vi "Main ACQ module2.vi"(8 "Update timer[ms]":u32=100, 9 "Master mailbox":T6, 11 "Module mailbox":T6) -> ()   [LabVIEW 2024, in "Lock-in module.lvlib"]
uses:
  Lock-in module.lvlib
  Messenger service/Data types/Mailbox address.ctl
  ctl/ACQ status.ctl
  <instrlib>/Zurich Instruments LabOne/Public/ziTypeHandle.ctl
  <instrlib>/Zurich Instruments LabOne/Public/Modules/ziTypeModHandle.ctl
  ctl/ACQ info.ctl
  ctl/Mode.ctl
  Messenger service/Data types/Module name.ctl
  ctl/MFLI_message for module.ctl
  ctl/MFLI_command enum.ctl
  ctl/MFLI parameters.ctl
  <instrlib>/Zurich Instruments LabOne/Public/Modules/ziTypeModEnum.ctl
  ctl/MFLI_parameter and value.ctl
  ctl/MFLI_node.ctl
  <instrlib>/Zurich Instruments LabOne/Public/Configure/ziSetValueDouble.vi
  <instrlib>/Zurich Instruments LabOne/Zurich Instruments LabOne.lvlib
  Messenger service/MessengerLib.lvlib
panel:
  out "time":u32
  out "Modulation amplitude [A]":dbl
  out "Multimeter name":string
  out "Multimeter port":refnum<visa-resource-name>
  out "Mode":T1=enum."Point"
  out "ACQ  status":T2={"Lock-in Handle"={"handleValid"=FALSE, "Conn"=0, "Path Prefix"="", "Handle"=0, "Connected"=FALSE, "Clockbase(s)"=0.0}, "Address"="DEV", "ModuleHandles"=[], "Lock-in info"={"In50"=FALSE, "InAC"=FALSE, "InDiff"=FALSE, "Out50"=FALSE, "OutEN"=FALSE, "OutF[Hz]"=0.0, "OutA[V]"=0.0, "DemEN"=FALSE, "Const[ms]"=0.0, "Order[-]"=0, "Phase [°]"=0.0}} {"ModuleHandles"."ModHandle" format="0x%08x"; "ModuleHandles"."Conn" format="0x%08x"; "Lock-in Handle"."Handle" format="0x%08x"; "Lock-in Handle"."Conn" format="0x%08x"}
  out "Selected Device":string
  out "Ended":bool
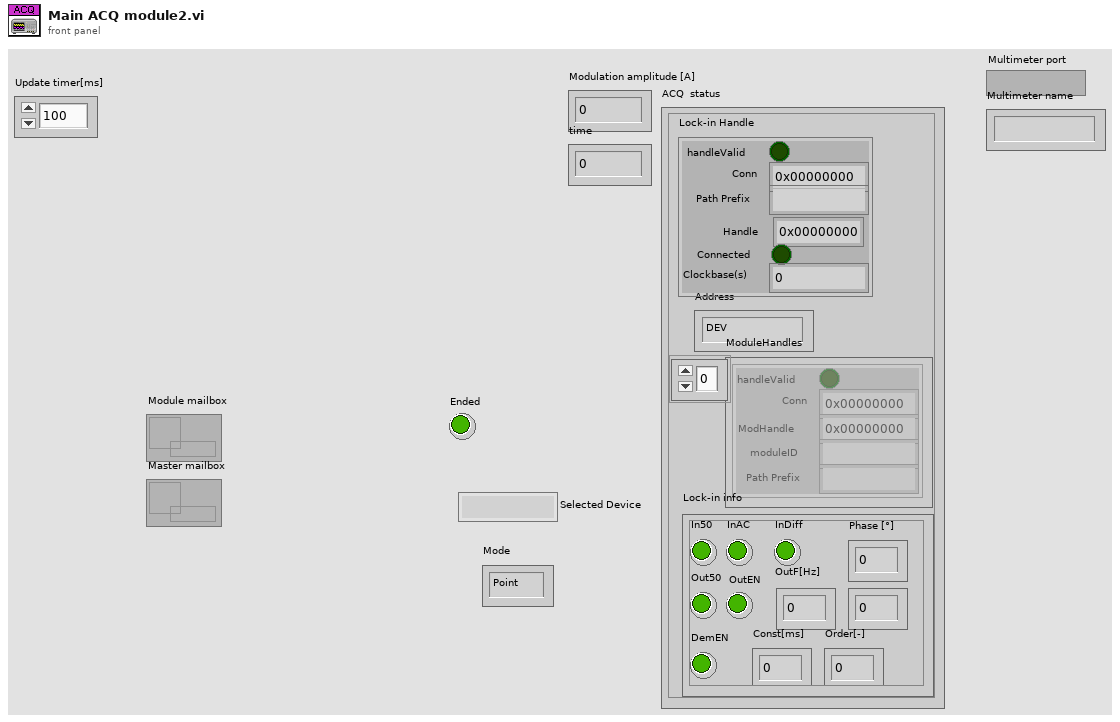
[diagram p1: front panel]
types:
  T1 = typedef "Lock-in module.lvlib/Mode.ctl" = enum16{"None", "Point", "Scope", "Both", "DAQ"}
  T2 = typedef "Lock-in module.lvlib/ACQ status.ctl" = cluster{"Lock-in Handle":T3, "Address":string, "ModuleHandles":T4[], "Lock-in info":T5}
  T3 = typedef "Zurich Instruments LabOne.lvlib/ziTypeHandle.ctl" = cluster{"handleValid":bool, "Conn":u64, "Path Prefix":string, "Handle":u64, "Connected":bool, "Clockbase(s)":dbl}
  T4 = typedef "Zurich Instruments LabOne.lvlib/ziTypeModHandle.ctl" = cluster{"handleValid":bool, "Conn":u64, "ModHandle":u64, "moduleID":string, "Path Prefix":string}
  T5 = typedef "Lock-in module.lvlib/ACQ info.ctl" = cluster{"In50":bool, "InAC":bool, "InDiff":bool, "Out50":bool, "OutEN":bool, "OutF[Hz]":dbl, "OutA[V]":dbl, "DemEN":bool, "Const[ms]":dbl, "Order[-]":i32, "Phase [°]":dbl}
  T6 = typedef "MessengerLib.lvlib/Mailbox address.ctl" = refnum<queue>
  T7 = typedef "Module name.ctl" = enum16{"Emty", "Magnet", "VTI", "Excitation", "Servo", "Acquisition", "Rotator", "Digitizer", "SMU2450", "Carousel", "Multimeter", "Tmp monitor", "Power monitor"}
  T8 = typedef "Lock-in module.lvlib/MFLI parameters.ctl" = cluster{"Filter order":dbl, "Time constant [ms]":dbl, "F_Mod [kHz]":dbl, "Amp_Mod [mV]":dbl, "Enable output":u16, "Phase [°]":dbl}
  T9 = typedef "Lock-in module.lvlib/MFLI_parameter and value.ctl" = cluster{"parameter":T10, "value":dbl}
  T10 = typedef "Lock-in module.lvlib/MFLI_node.ctl" = enum16{"None", "filter_order [-]", "filter_constant [ms]", "in_diff", "in_autorange", "in_imp50", "in_AC", "osc_freq [kHz]", "out_ampl [V]", "out_autorange", "out_imp50", "enable output", "enamble ampl", "scope_enable", "scope_rate", "scope_len", "scope_trigEn", "AuxOut_amplify", "Phase_deg", "AuxOut_select"}
  T11 = typedef "Lock-in module.lvlib/MFLI_command enum.ctl" = enum16{"Initialize", "Update", "Set parameters", "Set module", "Set individual parameters", "Get point", "Get array", "Disconnect", "End", "Ignore"}
  T12 = typedef "Zurich Instruments LabOne.lvlib/ziTypeModEnum.ctl" = u16
  T13 = typedef "Lock-in module.lvlib/MFLI_message for module.ctl" = cluster{"Command":T11, "Data":variant}
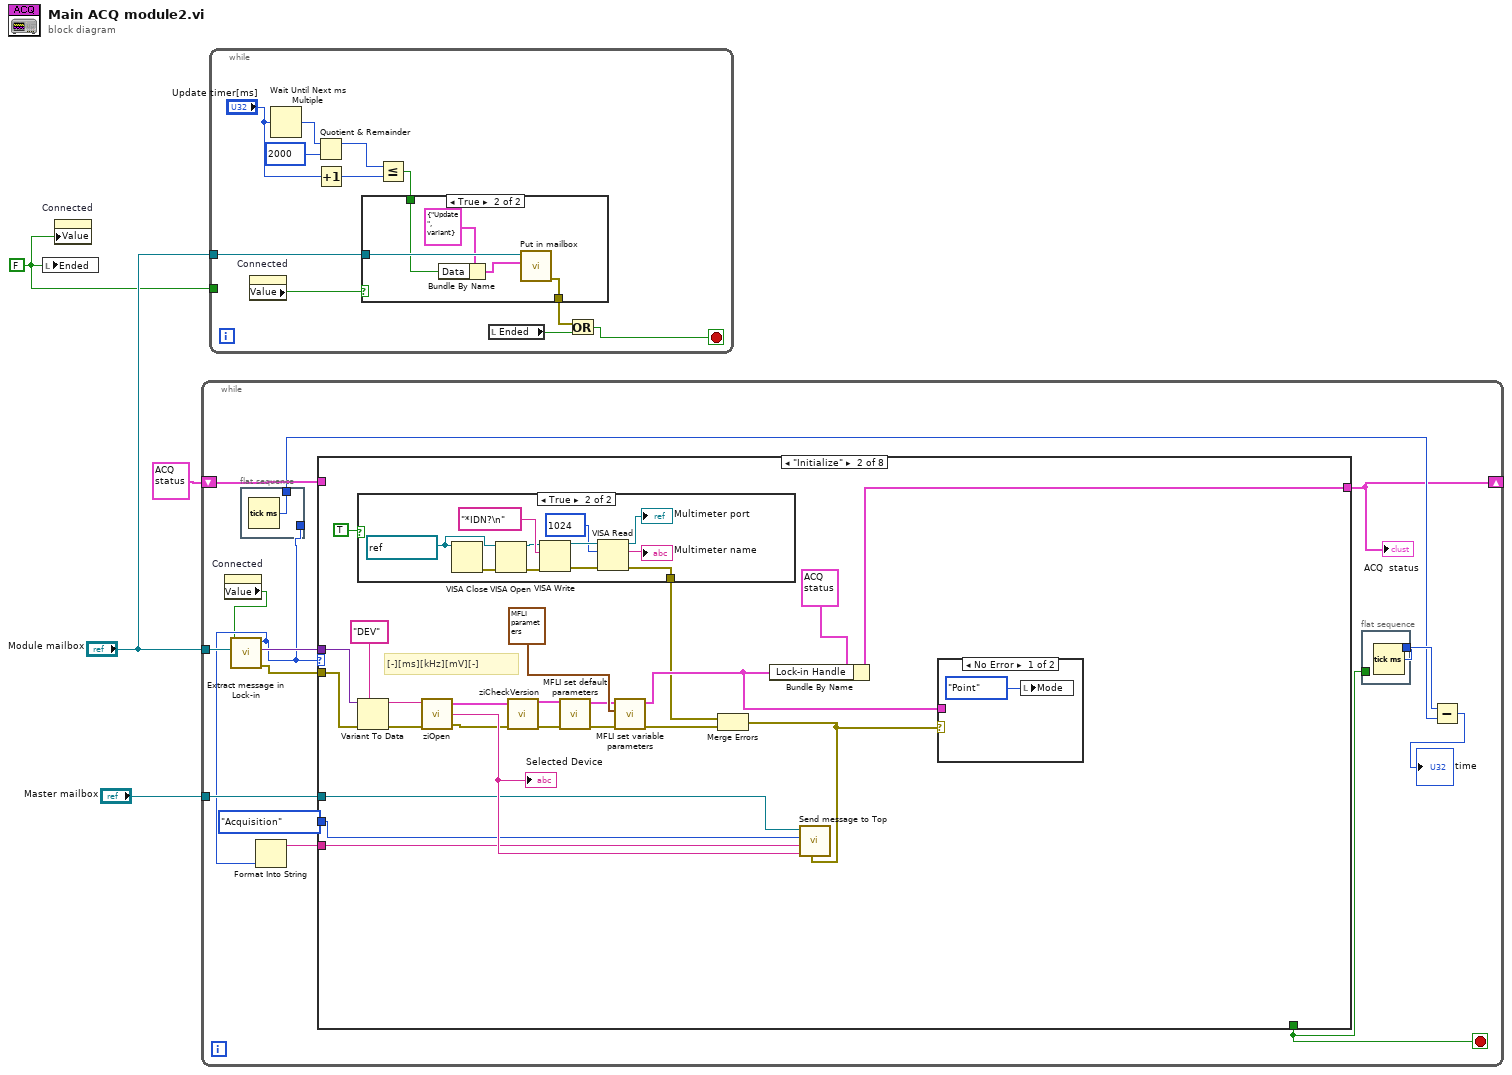
[diagram p0: block diagram]
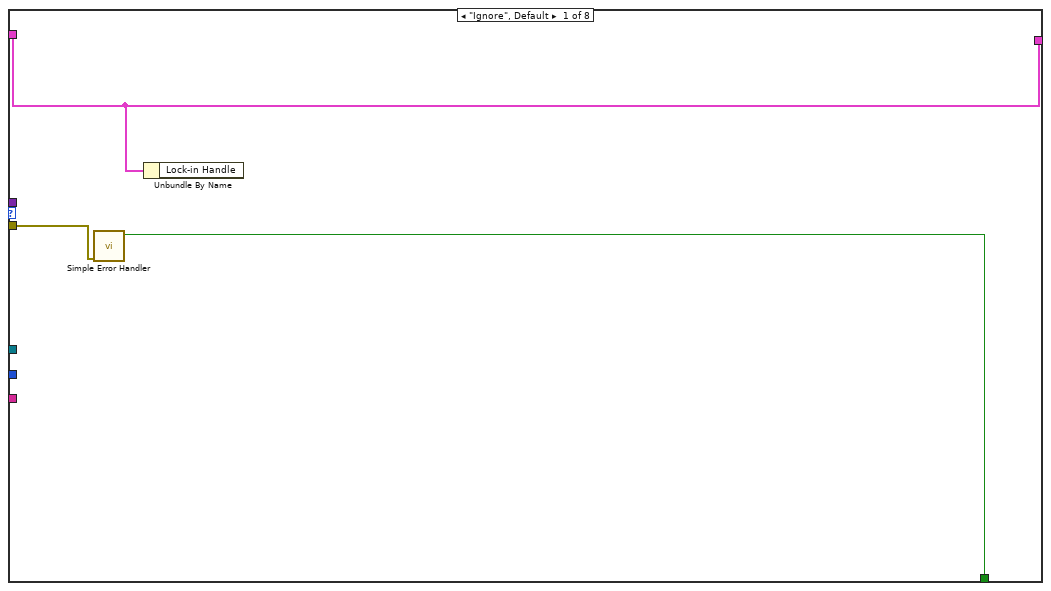
[diagram p2: hidden frame]
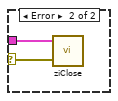
[diagram p4: hidden frame]
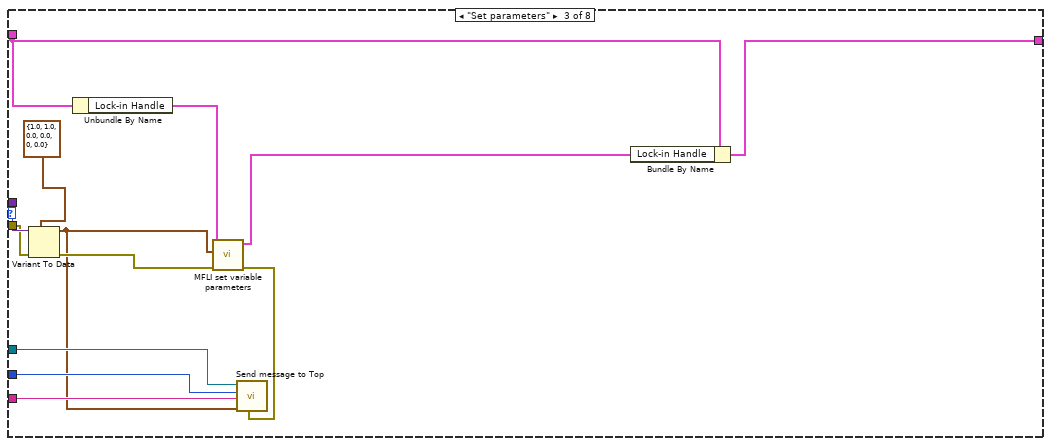
[diagram p5: hidden frame]
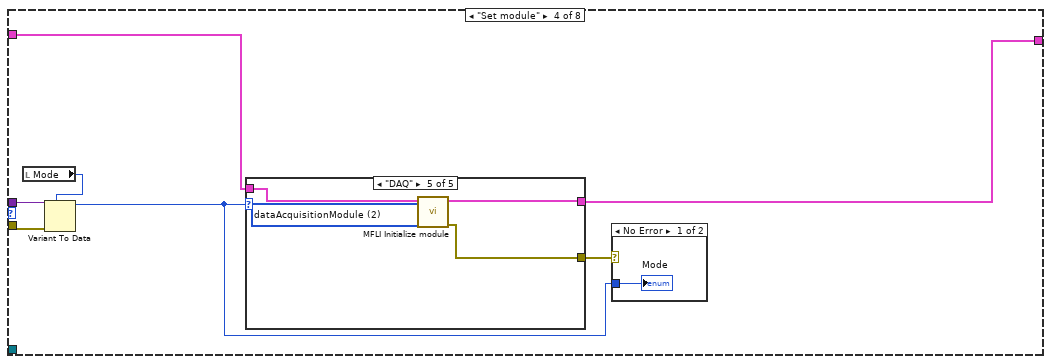
[diagram p6: hidden frame]
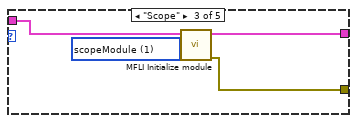
[diagram p10: hidden frame]
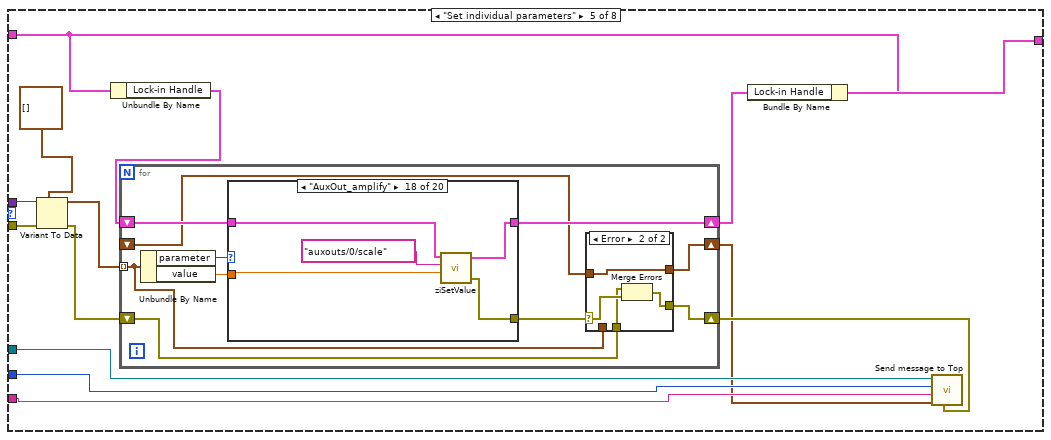
[diagram p12: hidden frame]
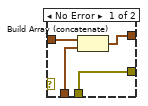
[diagram p13: hidden frame]
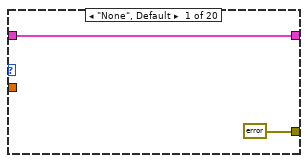
[diagram p14: hidden frame]
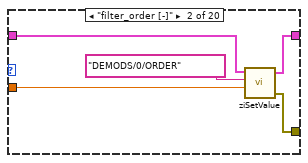
[diagram p15: hidden frame]
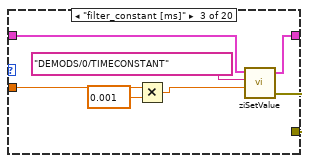
[diagram p16: hidden frame]
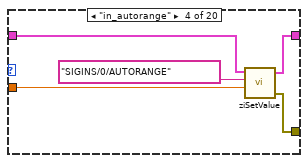
[diagram p17: hidden frame]
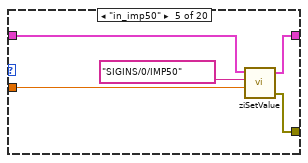
[diagram p18: hidden frame]
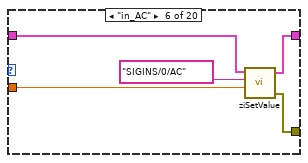
[diagram p19: hidden frame]
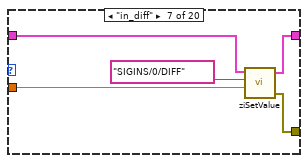
[diagram p20: hidden frame]
diagram:
  w1 = FALSE ("Initialized")
  n1 = local write "Ended"(w1) -> ()
  n2 = property on="Connected" class="Bool (strict)"("Value"=w1) -> ()  [unwired: 2 in, 2 out]
  n3 = while {
    tunnel: "Module mailbox" -> [w18]
    tunnel: "Master mailbox" -> [w17]
    shift-right: [w7] -> _
    shift-left: T2 {"Lock-in Handle"={"handleValid"=FALSE, "Conn"=0, "Path Prefix"="", "Handle"=0, "Connected"=FALSE, "Clockbase(s)"=0.0}, "Address"="DEV", "ModuleHandles"=[], "Lock-in info"={"In50"=FALSE, "InAC"=FALSE, "InDiff"=FALSE, "Out50"=FALSE, "OutEN"=FALSE, "OutF[Hz]"=0.0, "OutA[V]"=0.0, "DemEN"=FALSE, "Const[ms]"=0.0, "Order[-]"=0, "Phase [°]"=0.0}} -> [w14]
    stop <- w6 stop-if-true
    n4 = property on="Connected" class="Bool (strict)"() -> ("Value"=w5:bool)  [unwired: 2 in, 2 out]
    n5 = call "Extract message in Lock-in.vi"("Module mailbox"=w18, "Initialized?"=w5) -> ("error out"=w15:errorcluster, "Data"=w16:variant, "Command out"=w11:T11)  [unwired: 7 in]
    n6 = flat-sequence {
      tunnel: w11 -> [_]
      tunnel: [w20] -> w9
      frame #0 {
        n7 = Tick Count (ms)() -> (millisecond timer value=w20:u32)
      }
    }
    n8 = Format Into String(w11) -> (resulting string=w13:string)  [unwired: 3 in, 1 out]
    n9 = case shown="\"Initialize\"" w11 {
      tunnel: w17 -> [_ w39 w68 _ w96 w239 w283 w300]
      tunnel: w16 -> [_ w46 w73 w80 w106 w231 _ _]
      tunnel: w15 -> [w23 w44 w69 w79 w104 w243 w284 w301]
      tunnel: [w22 _ _ _ _ _ w274 FALSE] -> w6
      tunnel: [w21 w38 w70 w76 w103 w245 w276 w292] -> w7
      tunnel: w14 -> [w21 _ w71 w77 w101 w237 w285 w302]
      tunnel: w13 -> [_ w35 w67 _ w98 w234 w281 w297]
      tunnel: Module_name."Acquisition" ("Module") -> [_ w34 w66 _ w97 w236 w282 w298]
      frame "Ignore", Default {
        n10 = call <vilib>:"Simple Error Handler.vi"("error in (no error)"=w23) -> ("error?"=w22:bool)  [unwired: 4 in, 4 out]
        n11 = Unbundle By Name(w21) -> ()  [unwired: 1 out]
      }
      frame "Initialize" {
        # "[-][ms][kHz][mV][-]"
        n12 = case shown="True" TRUE {
          tunnel: [_ w49] -> w25
          frame False {
          }
          frame True {
            w56 = refnum<visa-resource-name> "COM6" ("VISA resource name")
            n13 = VISA Close(VISA resource name=w56) -> (error out=w57:errorcluster)  [unwired: 1 in]
            n14 = VISA Open(error in (no error)=w57, VISA resource name=w56) -> (VISA resource name=w51:refnum<visa-resource-name>, error out=w50:errorcluster)  [unwired: 3 in]
            n15 = VISA Write(VISA resource name=w51, write buffer="*IDN?\n", error in (no error)=w50) -> (VISA resource name out=w55:refnum<visa-resource-name>, error out=w54:errorcluster)  [unwired: 1 out]
            n16 = VISA Read(VISA resource name=w55, byte count=u32 1024, error in (no error)=w54) -> (VISA resource name out=→"Multimeter port":refnum<visa-resource-name>, read buffer=→"Multimeter name":string, error out=w49:errorcluster)  [unwired: 1 out]
          }
        }
        n17 = Variant To Data(error in=w44, type="DEV" ("Address"), Variant=w46) -> (data=w43:string, error out=w42:errorcluster)
        n18 = call <instrlib>:"ziOpen.vi"("Error In"=w42, "Address"=w43) -> ("Error Out"=w36:errorcluster, "Selected Device"=w40:string, "HandleOut"=w37:T3)  [unwired: 2 in]
        "Selected Device" <- w40
        n19 = call <instrlib>:"ziCheckVersion.vi"("Handle In"=w37, "Error In"=w36) -> ("Handle Out"=w32:T3, "Error Out"=w33:errorcluster)  [unwired: 11 in, 1 out]
        n20 = call "MFLI set default parameters.vi"("error in (no error)"=w33, "Lock-in Handle"=w32) -> ("Error Out"=w29:errorcluster, "Handle Out"=w30:T3)  [unwired: 8 in]
        n21 = call "MFLI set variable parameters.vi"("error in"=w29, "ACQ parameters"=T8 {"Filter order"=5.0, "Time constant [ms]"=50.0, "F_Mod [kHz]"=10.0, "Amp_Mod [mV]"=100.0, "Enable output"=0, "Phase [°]"=0.0}, "handle in"=w30) -> ("Error Out"=w28:errorcluster, "Handle Out"=w26:T3)  [unwired: 7 in]
        n22 = Merge Errors(w25, w28) -> (w27:errorcluster)
        n23 = Bundle By Name(cluster=T2 {"Lock-in Handle"={"handleValid"=FALSE, "Conn"=0, "Path Prefix"="", "Handle"=0, "Connected"=FALSE, "Clockbase(s)"=0.0}, "Address"="DEV", "ModuleHandles"=[], "Lock-in info"={"In50"=FALSE, "InAC"=FALSE, "InDiff"=FALSE, "Out50"=FALSE, "OutEN"=FALSE, "OutF[Hz]"=0.0, "OutA[V]"=0.0, "DemEN"=FALSE, "Const[ms]"=0.0, "Order[-]"=0, "Phase [°]"=0.0}}, "Lock-in Handle"=w26) -> (w38:T2)
        n24 = call "Send message to Top.vi"("Error in (no error)"=w27, "Data"=w40, "Response"=w35, "Module"=w34, "Mailbox address in"=w39) -> ()  [unwired: 5 in, 2 out]
        n25 = case shown="No Error" w27 {
          selector: w27 -> [_ w60]
          tunnel: w26 -> [_ w59]
          frame No Error {
            n26 = local write "Mode"(Mode."Point" ("Mode")) -> ()
          }
          frame Error {
            n27 = call <instrlib>:"ziClose.vi"("Error In"=w60, "Handle In"=w59) -> ()  [unwired: 2 in, 2 out]
          }
        }
      }
      frame "Set parameters" {
        n28 = Variant To Data(error in=w69, type=T8 {"Filter order"=1.0, "Time constant [ms]"=1.0, "F_Mod [kHz]"=0.0, "Amp_Mod [mV]"=0.0, "Enable output"=0, "Phase [°]"=0.0} ("ACQ parameters"), Variant=w73) -> (data=w61:T8, error out=w63:errorcluster)
        n29 = Unbundle By Name(w71) -> ("Lock-in Handle"=w64:T3)
        n30 = call "MFLI set variable parameters.vi"("error in"=w63, "ACQ parameters"=w61, "handle in"=w64) -> ("Error Out"=w65:errorcluster, "Handle Out"=w62:T3)  [unwired: 7 in]
        n31 = call "Send message to Top.vi"("Error in (no error)"=w65, "Data"=w61, "Response"=w67, "Module"=w66, "Mailbox address in"=w68) -> ()  [unwired: 5 in, 2 out]
        n32 = Bundle By Name(cluster=w71, "Lock-in Handle"=w62) -> (w70:T2)
      }
      frame "Set module" {
        n33 = local read "Mode"() -> (w78:T1)
        n34 = Variant To Data(error in=w79, type=w78, Variant=w80) -> (data=w74:T1)  [unwired: 1 out]
        n35 = case shown="\"DAQ\"" w74 {
          tunnel: w77 -> [w82 w83 w86 w88 w92]
          tunnel: [w82 w83 w85 w88 w90] -> w76
          tunnel: [_ _ w84 _ w89] -> w75
          frame "None", Default {
          }
          frame "Point" {
          }
          frame "Scope" {
            w87 = T12 1 items=["sweep", "scopeModule", "dataAcquisitionModule", "pidAdvisor", "awgModule", "impedanceModule", "multiDeviceSyncModule", "zoomFFT", "trigger", "deviceSettings", "record"] ("module Id")
            n36 = call "MFLI Initialize module.vi"("module Id"=w87, "ACQ  status in"=w86) -> ("Error Out"=w84:errorcluster, "ACQ  status out"=w85:T2)  [unwired: 8 in]
          }
          frame "Both" {
          }
          frame "DAQ" {
            w91 = T12 2 items=["sweep", "scopeModule", "dataAcquisitionModule", "pidAdvisor", "awgModule", "impedanceModule", "multiDeviceSyncModule", "zoomFFT", "trigger", "deviceSettings", "record"] ("module Id")
            n37 = call "MFLI Initialize module.vi"("module Id"=w91, "ACQ  status in"=w92) -> ("Error Out"=w89:errorcluster, "ACQ  status out"=w90:T2)  [unwired: 8 in]
          }
        }
        n38 = case shown="No Error" w75 {
          tunnel: w74 -> [w81 _]
          frame No Error {
            "Mode" <- w81
          }
          frame Error {
          }
        }
      }
      frame "Set individual parameters" {
        n39 = Variant To Data(error in=w104, type=T9[] [] ("Array"), Variant=w106) -> (data=w99:T9[], error out=w94:errorcluster)
        n40 = Unbundle By Name(w101) -> ("Lock-in Handle"=w102:T3)
        n41 = for {
          tunnel: w99 -> [w109] mode=indexing
          shift-right: [w115] -> w100
          shift-left: w102 -> [w116]
          shift-right: [w111] -> w95
          shift-left: w94 -> [w110]
          shift-right: [w108] -> w93
          shift-left: _ -> [w107]
          n42 = Unbundle By Name(w109) -> ("parameter"=w113:T10, "value"=w114:dbl)
          n43 = case shown="\"AuxOut_amplify\"" w113 {
            tunnel: w116 -> [w126 w131 w138 w143 w148 w153 w158 w165 w170 w175 w180 w185 w190 w195 w198 w205 w208 w213 w218 w223]
            tunnel: [w126 w130 w137 w142 w147 w152 w157 w164 w169 w174 w179 w184 w189 w194 w199 w204 w209 w214 w219 w224] -> w115
            tunnel: w114 -> [_ w129 w136 w141 w146 w151 w156 w161 w168 w173 w178 w183 w188 w192 w197 w203 w207 w212 w217 w222]
            tunnel: [errorcluster {"status"=FALSE, "code"=0, "source"=""} ("Error Out") w127 w134 w139 w144 w149 w154 w163 w166 w171 w176 w181 w186 w193 w200 w201 w210 w215 w220 w225] -> w112
            frame "None", Default {
            }
            frame "filter_order [-]" {
              n44 = call-poly <instrlib>:"ziSetValue.vi"("Value"=w129, "Path"="DEMODS/0/ORDER", "Handle In"=w131) -> ("Error Out"=w127:errorcluster, "Handle Out"=w130:T3)  [unwired: 2 in]
            }
            frame "filter_constant [ms]" {
              n45 = Multiply(x=w136, y=0.001) -> (x*y=w133:dbl)
              n46 = call-poly <instrlib>:"ziSetValue.vi"("Value"=w133, "Path"="DEMODS/0/TIMECONSTANT", "Handle In"=w138) -> ("Error Out"=w134:errorcluster, "Handle Out"=w137:T3)  [unwired: 2 in]
            }
            frame "in_autorange" {
              n47 = call-poly <instrlib>:"ziSetValue.vi"("Value"=w141, "Path"="SIGINS/0/AUTORANGE", "Handle In"=w143) -> ("Error Out"=w139:errorcluster, "Handle Out"=w142:T3)  [unwired: 2 in]
            }
            frame "in_imp50" {
              n48 = call-poly <instrlib>:"ziSetValue.vi"("Value"=w146, "Path"="SIGINS/0/IMP50", "Handle In"=w148) -> ("Error Out"=w144:errorcluster, "Handle Out"=w147:T3)  [unwired: 2 in]
            }
            frame "in_AC" {
              n49 = call-poly <instrlib>:"ziSetValue.vi"("Value"=w151, "Path"="SIGINS/0/AC", "Handle In"=w153) -> ("Error Out"=w149:errorcluster, "Handle Out"=w152:T3)  [unwired: 2 in]
            }
            frame "in_diff" {
              n50 = call-poly <instrlib>:"ziSetValue.vi"("Value"=w156, "Path"="SIGINS/0/DIFF", "Handle In"=w158) -> ("Error Out"=w154:errorcluster, "Handle Out"=w157:T3)  [unwired: 2 in]
            }
            frame "osc_freq [kHz]" {
              n51 = Multiply(x=w161, y=1000.0) -> (x*y=w160:dbl)
              n52 = call-poly <instrlib>:"ziSetValue.vi"("Value"=w160, "Path"="OSCS/0/FREQ", "Handle In"=w165) -> ("Error Out"=w163:errorcluster, "Handle Out"=w164:T3)  [unwired: 2 in]
            }
            frame "out_ampl [V]" {
              n53 = call-poly <instrlib>:"ziSetValue.vi"("Value"=w168, "Path"="SIGOUTS/0/AMPLITUDES/1", "Handle In"=w170) -> ("Error Out"=w166:errorcluster, "Handle Out"=w169:T3)  [unwired: 2 in]
            }
            frame "out_autorange" {
              n54 = call-poly <instrlib>:"ziSetValue.vi"("Value"=w173, "Path"="SIGOUTS/0/AUTORANGE", "Handle In"=w175) -> ("Error Out"=w171:errorcluster, "Handle Out"=w174:T3)  [unwired: 2 in]
            }
            frame "out_imp50" {
              n55 = call-poly <instrlib>:"ziSetValue.vi"("Value"=w178, "Path"="SIGOUTS/0/IMP50", "Handle In"=w180) -> ("Error Out"=w176:errorcluster, "Handle Out"=w179:T3)  [unwired: 2 in]
            }
            frame "enable output" {
              n56 = call-poly <instrlib>:"ziSetValue.vi"("Value"=w183, "Path"="SIGOUTS/0/ON", "Handle In"=w185) -> ("Error Out"=w181:errorcluster, "Handle Out"=w184:T3)  [unwired: 2 in]
            }
            frame "enamble ampl" {
              n57 = call-poly <instrlib>:"ziSetValue.vi"("Value"=w188, "Path"="SIGOUTS/0/ENABLES/1", "Handle In"=w190) -> ("Error Out"=w186:errorcluster, "Handle Out"=w189:T3)  [unwired: 2 in]
            }
            frame "scope_enable" {
              n58 = call-poly <instrlib>:"ziSetValue.vi"("Value"=w192, "Path"="scopes/0/enable", "Handle In"=w195) -> ("Error Out"=w193:errorcluster, "Handle Out"=w194:T3)  [unwired: 2 in]
            }
            frame "scope_rate" {
              n59 = call-poly <instrlib>:"ziSetValue.vi"("Value"=w197, "Path"="scopes/0/time", "Handle In"=w198) -> ("Error Out"=w200:errorcluster, "Handle Out"=w199:T3)  [unwired: 2 in]
            }
            frame "scope_trigEn" {
              n60 = call-poly <instrlib>:"ziSetValue.vi"("Value"=w203, "Path"="SCOPES/0/TRIGENABLE", "Handle In"=w205) -> ("Error Out"=w201:errorcluster, "Handle Out"=w204:T3)  [unwired: 2 in]
            }
            frame "scope_len" {
              n61 = call-poly <instrlib>:"ziSetValue.vi"("Value"=w207, "Path"="scopes/0/length", "Handle In"=w208) -> ("Error Out"=w210:errorcluster, "Handle Out"=w209:T3)  [unwired: 2 in]
            }
            frame "AuxOut_amplify" {
              n62 = call-poly <instrlib>:"ziSetValue.vi"("Value"=w212, "Path"="auxouts/0/scale", "Handle In"=w213) -> ("Error Out"=w215:errorcluster, "Handle Out"=w214:T3)  [unwired: 2 in]
            }
            frame "Phase_deg" {
              n63 = call-poly <instrlib>:"ziSetValue.vi"("Value"=w217, "Path"="demods/1/phaseshift", "Handle In"=w218) -> ("Error Out"=w220:errorcluster, "Handle Out"=w219:T3)  [unwired: 2 in]
            }
            frame "AuxOut_select" {
              n64 = call-poly <instrlib>:"ziSetValue.vi"("Value"=w222, "Path"="auxouts/0/outputselect", "Handle In"=w223) -> ("Error Out"=w225:errorcluster, "Handle Out"=w224:T3)  [unwired: 2 in]
            }
          }
          n65 = case shown="Error" w112 {
            selector: w112 -> [_ w124]
            tunnel: [w120 w123] -> w111
            tunnel: w110 -> [w120 w122]
            tunnel: w109 -> [w118 _]
            tunnel: [w119 w121] -> w108
            tunnel: w107 -> [w117 w121]
            frame No Error {
              n66 = Build Array (concatenate)(w117, w118) -> (w119:T9[])
            }
            frame Error {
              n67 = Merge Errors(w122, w124) -> (w123:errorcluster)
            }
          }
        }
        n68 = Bundle By Name(cluster=w101, "Lock-in Handle"=w100) -> (w103:T2)
        n69 = call "Send message to Top.vi"("Error in (no error)"=w95, "Data"=w93, "Response"=w98, "Module"=w97, "Mailbox address in"=w96) -> ()  [unwired: 5 in, 2 out]
      }
      frame "Update" {
        n70 = Unbundle By Name(w237) -> ("Lock-in info"=w228:T5, "ModuleHandles"=w227:T4[], "Lock-in Handle"=w244:T3)
        n71 = Variant To Data(error in=w243, type=TRUE, Variant=w231) -> (data=w229:bool, error out=w232:errorcluster)
        n72 = case shown="True" w229 {
          tunnel: w244 -> [w249 w259]
          tunnel: [w249 w258] -> w240
          tunnel: w239 -> [w246 w257]
          tunnel: [w247 w255] -> w238
          tunnel: w236 -> [_ w254]
          tunnel: [w246 w253] -> w235
          tunnel: w234 -> [_ w252]
          tunnel: [w248 w251] -> w233
          tunnel: w232 -> [w247 w250]
          tunnel: w228 -> [w248 _]
          frame False {
          }
          frame True {
            n73 = call "Lock-in update.vi"("error in (no error)"=w250, "Lock-in Handle"=w259) -> ("error out"=w256:errorcluster, "Lock-in info"=w251:T5, "Handle Out"=w258:T3)  [unwired: 7 in]
            n74 = call "Send message to Top.vi"("Error in (no error)"=w256, "Data"=w251, "Response"=w252, "Module"=w254, "Mailbox address in"=w257) -> ("Error out"=w255:errorcluster, "Mailbox address out"=w253:T6)  [unwired: 5 in]
          }
        }
        n75 = case shown="True" w229 {
          tunnel: w236 -> [_ w265]
          tunnel: w235 -> [_ w262]
          frame False {
          }
          frame True {
            n76 = local read "Multimeter port"() -> (w273:refnum<visa-resource-name>)
            n77 = VISA Write(VISA resource name=w273, write buffer="READ?\n") -> (VISA resource name out=w272:refnum<visa-resource-name>, error out=w261:errorcluster)  [unwired: 1 in, 1 out]
            n78 = VISA Read(VISA resource name=w272, byte count=u32 1024, error in (no error)=w261) -> (read buffer=w270:string, error out=w260:errorcluster)  [unwired: 2 out]
            n79 = String Subset(string=w270, length (rest)=11 ("length (rest)")) -> (substring=w271:string)  [unwired: 1 in]
            n80 = Scan Value(string=w271, format string="%g") -> (value=w264:dbl)  [unwired: 1 in, 1 out]
            "Modulation amplitude [A]" <- w264
            n81 = call "Send message to Top.vi"("Error in (no error)"=w260, "Data"=w264, "Response"="Get ModA", "Module"=w265, "Mailbox address in"=w262) -> ()  [unwired: 5 in, 2 out]
          }
        }
        n82 = local read "Mode"() -> (w241:T1)
        n83 = call "MFLI read data.vi"("Module"=w236, "ModuleHandles in"=w227, "error in (no error)"=w238, "lock-in handle in"=w240, "Mode"=w241, "Queue in"=w235) -> ("ModuleHandles out"=w226:T4[], "Handle Out out"=w242:T3)  [unwired: 4 in]
        n84 = Bundle By Name(cluster=w237, "Lock-in Handle"=w242, "ModuleHandles"=w226, "Lock-in info"=w233) -> (w245:T2)
      }
      frame "End" {
        w274 = TRUE
        n85 = Unbundle By Name(w285) -> ("Lock-in Handle"=w278:T3)
        n86 = local read "Mode"() -> (w280:T1)
        n87 = case shown="\"Scope\", \"Both\"" w280 {
          tunnel: w278 -> [w287 w290]
          tunnel: [w287 w288] -> w279
          frame "None", Default {
          }
          frame "Scope", "Both" {
            n88 = call <instrlib>:"ziUnSubscribe.vi"("Path (\"/\")"="scopes/0/wave" ("Path"), "Handle in"=w290) -> ("Handle out"=w288:T3)  [unwired: 2 in, 1 out]
          }
        }
        n89 = call <instrlib>:"ziClose.vi"("Error In"=w284, "Handle In"=w279) -> ("Handle Out"=w275:T3)  [unwired: 2 in, 1 out]
        n90 = call "Send message to Top.vi"("Data"=w275, "Response"=w281, "Module"=w282, "Mailbox address in"=w283) -> ()  [unwired: 6 in, 2 out]
        n91 = case shown="False" TRUE {
          frame False {
          }
          frame True {
            n92 = local read "Multimeter port"() -> (w286:refnum<visa-resource-name>)
            n93 = VISA Close(VISA resource name=w286) -> ()  [unwired: 1 in, 1 out]
          }
        }
        n94 = Bundle By Name(cluster=w285, "Lock-in Handle"=w275) -> (w276:T2)
        "Ended" <- w274
      }
      frame "Disconnect" {
        n95 = Unbundle By Name(w302) -> ("Lock-in Handle"=w294:T3)
        n96 = local read "Mode"() -> (w296:T1)
        n97 = case shown="\"Scope\", \"Both\"" w296 {
          tunnel: w294 -> [w305 w308]
          tunnel: [w305 w306] -> w295
          frame "None", Default {
          }
          frame "Scope", "Both" {
            n98 = call <instrlib>:"ziUnSubscribe.vi"("Path (\"/\")"="scopes/0/wave" ("Path"), "Handle in"=w308) -> ("Handle out"=w306:T3)  [unwired: 2 in, 1 out]
          }
        }
        n99 = call <instrlib>:"ziClose.vi"("Error In"=w301, "Handle In"=w295) -> ("Handle Out"=w291:T3)  [unwired: 2 in, 1 out]
        n100 = call "Send message to Top.vi"("Data"=w291, "Response"=w297, "Module"=w298, "Mailbox address in"=w300) -> ()  [unwired: 6 in, 2 out]
        n101 = case shown="True" TRUE {
          frame False {
          }
          frame True {
            n102 = local read "Multimeter port"() -> (w304:refnum<visa-resource-name>)
            n103 = VISA Close(VISA resource name=w304) -> ()  [unwired: 1 in, 1 out]
          }
        }
        n104 = local write "Ended"(FALSE ("Initialized")) -> ()
        n105 = Bundle By Name(cluster=w302, "Lock-in Handle"=w291) -> (w292:T2)
      }
    }
    "ACQ  status" <- w7
    n106 = flat-sequence {
      tunnel: [w19] -> w10
      tunnel: w6 -> [_]
      frame #0 {
        n107 = Tick Count (ms)() -> (millisecond timer value=w19:u32)
      }
    }
    n108 = Subtract(x=w10, y=w9) -> (x-y=→"time":u32)
  }
  n109 = while {
    tunnel: "Module mailbox" -> [w319]
    tunnel: w1 -> [_]
    stop <- w310 stop-if-true
    n110 = property on="Connected" class="Bool (strict)"() -> ("Value"=w312:bool)  [unwired: 2 in, 2 out]
    n111 = Wait Until Next ms Multiple(millisecond multiple="Update timer[ms]") -> (millisecond timer value=w318:u32)
    n112 = Quotient & Remainder(x=w318, y=u32 2000) -> (x-y*floor(x/y)=w316:u32)  [unwired: 1 out]
    n113 = Increment(x="Update timer[ms]") -> (x+1=w313:u32)
    n114 = Less Or Equal?(x=w316, y=w313) -> (x <= y?=w314:bool)
    n115 = case shown="True" w312 {
      tunnel: w319 -> [_ w324]
      tunnel: w314 -> [_ w321]
      tunnel: [_ w320] -> w311
      frame False {
      }
      frame True {
        n116 = Bundle By Name(cluster=T13 {"Command"=enum."Update", "Data"=variant} ("MSG for  ACQ"), "Data"=w321) -> (w322:T13)
        n117 = call "Put in mailbox.vi"("Message"=w322, "Queue in"=w324) -> ("error out"=w320:errorcluster)  [unwired: 7 in, 2 out]
      }
    }
    n118 = local read "Ended"() -> (w309:bool)
    n119 = Or(x=w311, y=w309) -> (x .or. y?=w310:bool)
  }
